vi "PWM_dutyCycle_LED.vi"() -> ()   [LabVIEW 2020]
uses:
  <vilib>/LabVIEW Interface for Arduino/Type Defs/Board Type.ctl
  <vilib>/LabVIEW Interface for Arduino/Type Defs/Pin Mode.ctl
  <vilib>/LabVIEW Interface for Arduino/LabVIEW Interface for Arduino.lvlib
panel:
  out "Waveform Chart":dbl(graph)
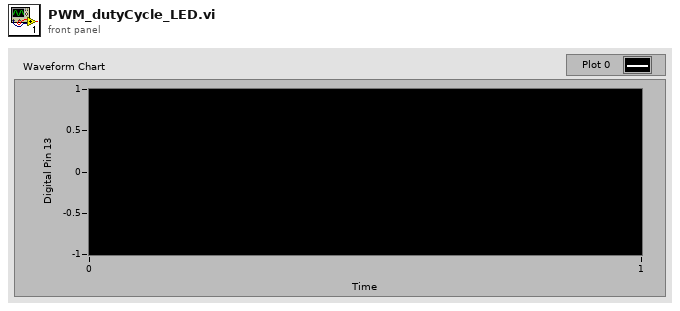
[diagram p1: front panel]
types:
  T1 = typedef "LabVIEW Interface for Arduino.lvlib/Pin Mode.ctl" = enum8{"Input", "Output"}
  T2 = typedef "LabVIEW Interface for Arduino.lvlib/Board Type.ctl" = enum16{"Uno", "Dimuelanove w/Atmega 328", "Mega 2560"}
  T3 = typedef "LabVIEW Interface for Arduino.lvlib/Arduino Resource.ctl" = cluster{"VISA resource":refnum<visa-resource-name>, "Board Type":T2, "Connection Type":enum8{"USB / Serial"}, "Bytes Per Packet (15)":u8}
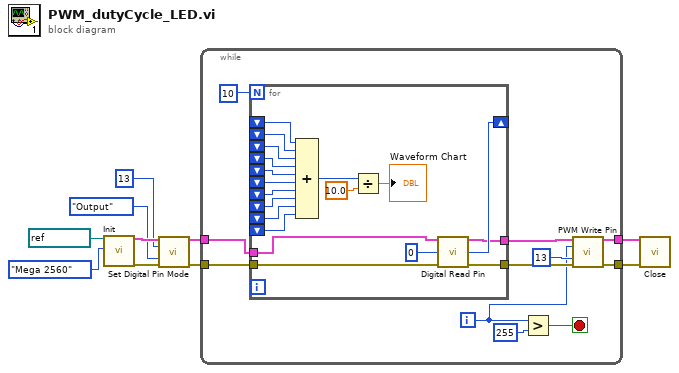
[diagram p0: block diagram]
diagram:
  n1 = call <vilib>:"Init.vi"("VISA resource"=refnum<visa-resource-name> "COM5", "Board Type (Uno)"=Board_Type."Mega 2560") -> ("Arduino Resource"=w8:T3, "error out"=w3:errorcluster)  [unwired: 16 in]
  n2 = call <vilib>:"Set Digital Pin Mode.vi"("Arduino Resource"=w8, "Digital I/O Pin"=u8 13, "Pin Mode (Input)"=Pin_Mode."Output", "error in"=w3) -> ("Arduino Resource"=w5:T3, "error out"=w4:errorcluster)  [unwired: 10 in]
  n3 = while {
    tunnel: w5 -> [w20]
    tunnel: w4 -> [w19]
    tunnel: [w15] -> w2
    tunnel: [w14] -> w1
    i -> [w13]
    stop <- w11 stop-if-true
    n4 = for {
      N: 10 -> [_]
      tunnel: [w40] -> w17
      tunnel: [w23] -> w18
      tunnel: w20 -> [w39]
      tunnel: w19 -> [w38]
      shift-right: [w37] -> _
      shift-left: _ -> [w36]
      shift-left: _ -> [w35]
      shift-left: _ -> [w34]
      shift-left: _ -> [w33]
      shift-left: _ -> [w32]
      shift-left: _ -> [w31]
      shift-left: _ -> [w30]
      shift-left: _ -> [w29]
      shift-left: _ -> [w28]
      shift-left: _ -> [w27]
      n5 = Compound Arithmetic op=ADD(w36, w35, w34, w33, w32, w31, w30, w29, w28, w27) -> (w25:u8)
      n6 = Divide(x=w25, y=10.0) -> (x/y=→"Waveform Chart":dbl)
      n7 = call <vilib>:"Digital Read Pin.vi"("Arduino Resource"=w39, "Digital I/O Pin (0)"=u8 0, "error in"=w38) -> ("Arduino Resource"=w23:T3, "Value"=w37:u8, "error out"=w40:errorcluster)  [unwired: 10 in]
    }
    n8 = Greater?(x=w13, y=255) -> (0:w11:bool)
    n9 = call <vilib>:"PWM Write Pin.vi"("Arduino Resource"=w18, "Duty Cycle (0 - 255)"=w13, "PWM Pin (3)"=u8 13, "error in"=w17) -> ("Arduino Resource"=w15:T3, "error out"=w14:errorcluster)  [unwired: 10 in]
  }
  n10 = call <vilib>:"Close.vi"("Arduino Resource"=w2, "error in"=w1) -> ()  [unwired: 13 in, 1 out]
